vi "Configure Channels.vi"(8 "error in":errorcluster, 11 "Scope PXI CFG in":refnum<class "Scope PXI CFG.lvclass">) -> (0 "error out":errorcluster, 3 "Scope PXI CFG out":refnum<class "Scope PXI CFG.lvclass">)   [LabVIEW 2023, in "Scope.lvlib" / "Scope PXI.lvlib" / "Scope PXI CFG.lvclass"]
uses:
  Scope PXI CFG.lvclass
  D:/git/HAL/Configuration Base/Configuration Base.lvclass
  <instrlib>/niScope/Controls/niScope vertical coupling.ctl
  Scope PXI CFG.lvclass/Scope PXI CFG.ctl
  Configuration Base/Configuration Base.lvclass/Configuration Base.ctl
  853bd4bf-b846-4392-aaec-2eb0df7c15c1.vi
  fc1a35be-1af8-4cb9-88ab-84357ec016c8.vi
  c0a7b2a4-d6e1-41c5-8fb1-93d513341217.vi
  d2234409-928f-4ed9-b693-2867399abf4a.vi
  1e64d3fa-bcbf-4fb7-97e9-849c0281c434.vi
  2f0dfe3b-727d-435f-a334-361c3472aed8.vi
  a8bb4bbf-f82b-4e58-9fc0-885d6d8595a7.vi
  2afd0b27-f59c-4e4c-ab34-d1b063ee1579.vi
  46d73ebe-6710-4003-86ab-c95650fc7a2a.vi
  88285a36-7fea-47d7-9b3a-47c90033b7a9.vi
  <vilib>/JDP Science/JSONtext/Find Item.vi
  <vilib>/JDP Science/JSONtext/Next JSON Value.vi
  <vilib>/JDP Science/JSONtext/String Subset.vi
  <vilib>/JDP Science/JSONtext/Parsing/Advance past next JSON Value (inlined COPY).vi
  <vilib>/JDP Science/JSONtext/Parsing/Advance past whitespace.vi
  <vilib>/JDP Science/JSONtext/Parsing/Advance past String.vi
  <vilib>/JDP Science/JSONtext/Parsing/Advance past Number.vi
  <vilib>/JDP Science/JSONtext/Parsing/Advance past Line Ending.vi
  <vilib>/JDP Science/JSONtext/Parsing/Parse Full Path or Item Name.vi
  <vilib>/JDP Science/JSONtext/Parsing/Advance past Array.vi
  <vilib>/JDP Science/JSONtext/Parsing/Advance past Object.vi
  <vilib>/JDP Science/JSONtext/support/Error Cluster From Code.vi
  <vilib>/JDP Science/JSONtext/Offset/Find Item Locations by Path.vi
  <vilib>/JDP Science/JSONtext/JSON text to Variant.vi
  <vilib>/Utility/error.llb/Error Cluster From Error Code.vi
  <vilib>/JDP Science/JSONtext/LVClass Serializer/JSONtext LVClass Serializer.lvclass
  <vilib>/ErrorRing/Error Ring.xnode
  Configuration Base/Configuration Base.lvclass
panel:
  out "vertical coupling":T1=1 caption="vertical coupling (DC)" items=["AC", "DC", "Ground"]
  out "input impedance":u32(ring)=2 items=["1 mega ohm"=0, "50 ohms"=2]
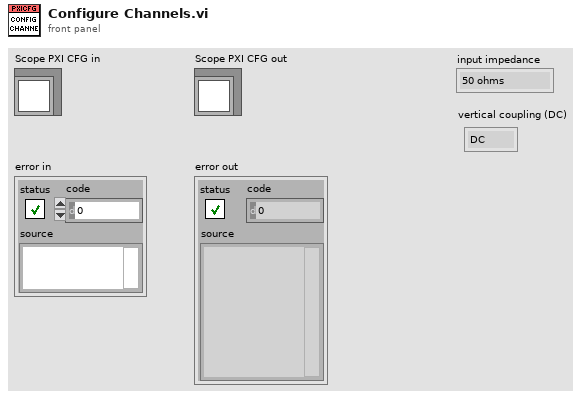
[diagram p1: front panel]
types:
  T1 = typedef "niScope vertical coupling.ctl" = i32
  T2 = typedef "LVStringsAndValuesArrayTypeDef_U32.ctl" = cluster{"String":string, "Value":u32}[]
  T3 = typedef "LVStringsAndValuesArrayTypeDef_I32.ctl" = cluster{"String":string, "Value":i32}[]
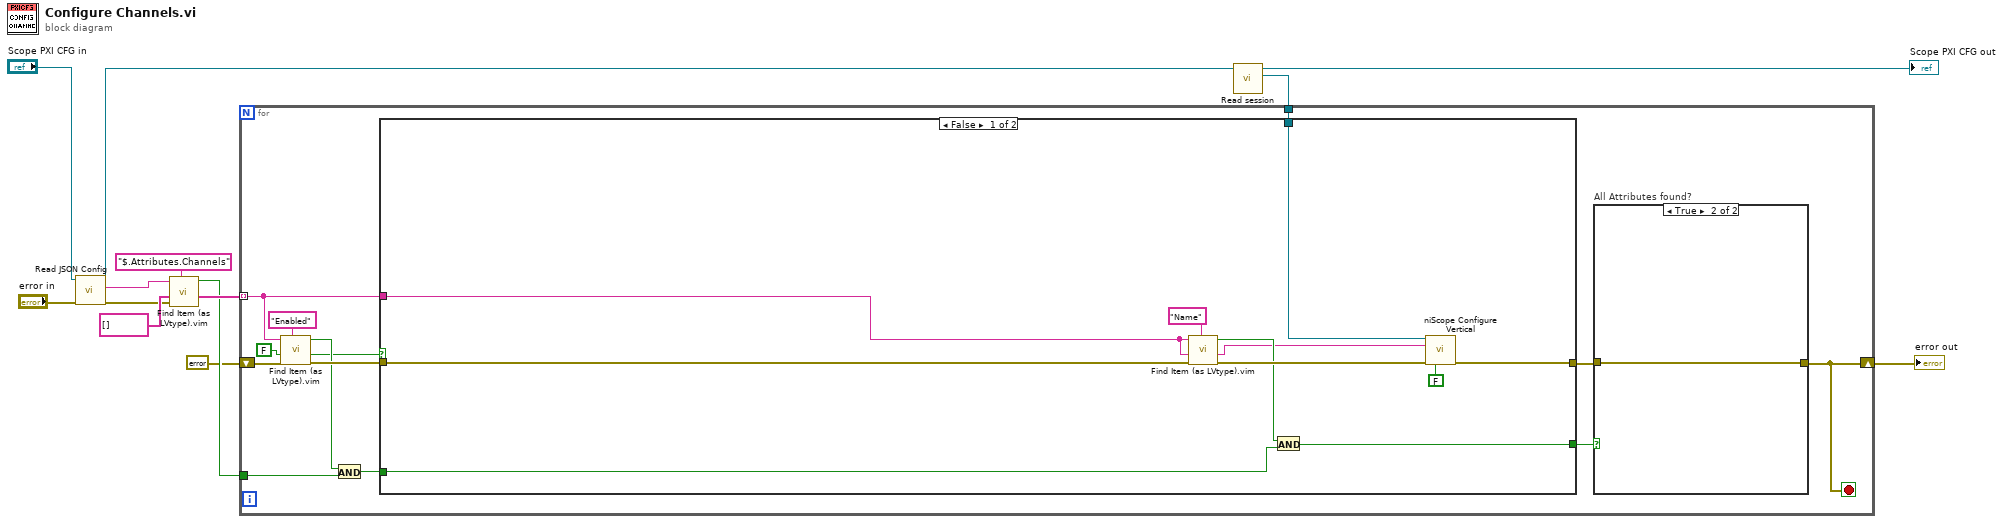
[diagram p0: block diagram]
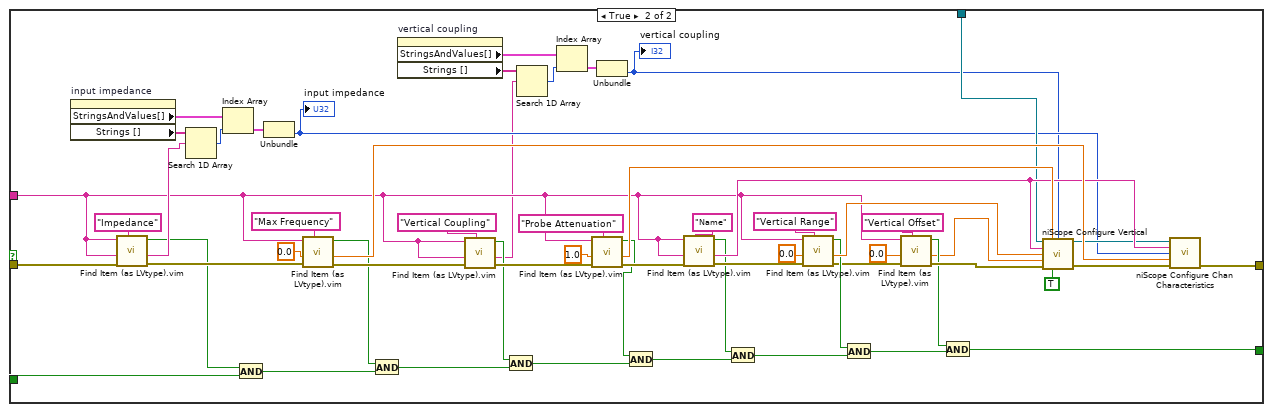
[diagram p2: hidden frame]
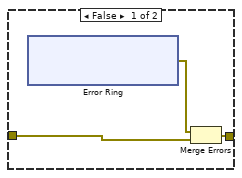
[diagram p3: hidden frame]
diagram:
  n1 = call "Read JSON Config.vi"("error in"="error in", "object in"="Scope PXI CFG in") -> ("error out"=w10:errorcluster, "<JSON>Config"=w11:string, "object out"=w2:refnum<class "Scope PXI CFG.lvclass">)  [unwired: 7 in]
  n2 = call "Find Item (as LVtype).vim"("$Path or Item Name"="$.Attributes.Channels", "error in (no error)"=w10, "Data Type and Default Value"=string[] [], "JSON"=w11) -> ("Data"=w9:string[], "Found"=w7:bool)  [unwired: 4 in, 2 out]
  n3 = call "Read session.vi"("Scope PXI CFG in"=w2) -> ("session"=w8:refnum<k15>, "Scope PXI CFG out"=→"Scope PXI CFG out":refnum<class "Scope PXI CFG.lvclass">)  [unwired: 8 in, 1 out]
  n4 = for {
    shift-right: [w14] -> w4
    shift-left: errorcluster {"status"=FALSE, "code"=0, "source"=""} ("error out") -> [w26]
    tunnel: w9 -> [w20] mode=indexing
    tunnel: w8 -> [w19]
    tunnel: w7 -> [w18]
    stop <- w14 stop-if-true
    n5 = call "Find Item (as LVtype).vim"("$Path or Item Name"="Enabled", "error in (no error)"=w26, "Data Type and Default Value"=FALSE, "JSON"=w20) -> ("error out"=w25:errorcluster, "Data"=w17:bool, "Found"=w22:bool)  [unwired: 4 in, 1 out]
    n6 = And(x=w22, y=w18) -> (x .and. y?=w23:bool)
    n7 = case shown="False" w17 {
      tunnel: [w27 w94] -> w16
      tunnel: w25 -> [w33 w77]
      tunnel: w23 -> [w37 w76]
      tunnel: w20 -> [w34 w44]
      tunnel: w19 -> [w28 w59]
      tunnel: [w31 w56] -> w15
      frame False {
        n8 = call "Find Item (as LVtype).vim"("$Path or Item Name"="Name", "error in (no error)"=w33, "Data Type and Default Value"=w34, "JSON"=w34) -> ("error out"=w32:errorcluster, "Data"=w29:string, "Found"=w30:bool)  [unwired: 4 in, 1 out]
        n9 = And(x=w30, y=w37) -> (x .and. y?=w31:bool)
        n10 = call <instrlib>:"niScope Configure Vertical.vi"("instrument handle"=w28, "channels"=w29, "error in"=w32, "channel enabled"=FALSE) -> ("error out"=w27:errorcluster)  [unwired: 10 in, 1 out]
      }
      frame True {
        n11 = property on="input impedance" class="Ring (strict)"() -> ("StringsAndValues[]"=w49:T2, "Strings []"=w48:string[])  [unwired: 2 in, 2 out]
        n12 = call "Find Item (as LVtype).vim"("$Path or Item Name"="Impedance", "error in (no error)"=w77, "Data Type and Default Value"=w44, "JSON"=w44) -> ("error out"=w93:errorcluster, "Data"=w47:string, "Found"=w46:bool)  [unwired: 4 in, 1 out]
        n13 = Search 1D Array(1D array=w48, element=w47) -> (index of element=w50:i32)  [unwired: 1 in]
        n14 = Index Array(array=w49, index=w50) -> (element=w51:cluster{"String":string, "Value":u32})
        n15 = And(x=w46, y=w76) -> (x .and. y?=w74:bool)
        n16 = Unbundle(w51) -> ("Value"=w45:u32)  [unwired: 1 out]
        "input impedance" <- w45
        n17 = call "Find Item (as LVtype).vim"("$Path or Item Name"="Max Frequency", "error in (no error)"=w93, "Data Type and Default Value"=0.0, "JSON"=w44) -> ("error out"=w90:errorcluster, "Data"=w85:dbl, "Found"=w75:bool)  [unwired: 4 in, 1 out]
        n18 = And(x=w75, y=w74) -> (x .and. y?=w72:bool)
        n19 = property on="vertical coupling" class="Ring (strict)"() -> ("StringsAndValues[]"=w40:T3, "Strings []"=w43:string[])  [unwired: 2 in, 2 out]
        n20 = call "Find Item (as LVtype).vim"("$Path or Item Name"="Vertical Coupling", "error in (no error)"=w90, "Data Type and Default Value"=w44, "JSON"=w44) -> ("error out"=w86:errorcluster, "Data"=w41:string, "Found"=w73:bool)  [unwired: 4 in, 1 out]
        n21 = And(x=w73, y=w72) -> (x .and. y?=w70:bool)
        n22 = Search 1D Array(1D array=w43, element=w41) -> (index of element=w42:i32)  [unwired: 1 in]
        n23 = Index Array(array=w40, index=w42) -> (element=w39:cluster{"String":string, "Value":i32})
        n24 = call "Find Item (as LVtype).vim"("$Path or Item Name"="Probe Attenuation", "error in (no error)"=w86, "Data Type and Default Value"=1.0, "JSON"=w44) -> ("error out"=w82:errorcluster, "Data"=w84:dbl, "Found"=w71:bool)  [unwired: 4 in, 1 out]
        n25 = Unbundle(w39) -> ("Value"=w38:i32)  [unwired: 1 out]
        "vertical coupling" <- w38
        n26 = And(x=w71, y=w70) -> (x .and. y?=w68:bool)
        n27 = call "Find Item (as LVtype).vim"("$Path or Item Name"="Name", "error in (no error)"=w82, "Data Type and Default Value"=w44, "JSON"=w44) -> ("error out"=w81:errorcluster, "Data"=w80:string, "Found"=w69:bool)  [unwired: 4 in, 1 out]
        n28 = And(x=w69, y=w68) -> (x .and. y?=w66:bool)
        n29 = call "Find Item (as LVtype).vim"("$Path or Item Name"="Vertical Range", "error in (no error)"=w81, "Data Type and Default Value"=0.0, "JSON"=w44) -> ("error out"=w63:errorcluster, "Data"=w78:dbl, "Found"=w67:bool)  [unwired: 4 in, 1 out]
        n30 = And(x=w67, y=w66) -> (x .and. y?=w65:bool)
        n31 = call "Find Item (as LVtype).vim"("$Path or Item Name"="Vertical Offset", "error in (no error)"=w63, "Data Type and Default Value"=0.0, "JSON"=w44) -> ("error out"=w62:errorcluster, "Data"=w60:dbl, "Found"=w61:bool)  [unwired: 4 in, 1 out]
        n32 = And(x=w61, y=w65) -> (x .and. y?=w56:bool)
        n33 = call <instrlib>:"niScope Configure Vertical.vi"("instrument handle"=w59, "probe attenuation"=w84, "vertical coupling"=w38, "channels"=w80, "vertical range"=w78, "vertical offset"=w60, "error in"=w62, "channel enabled"=TRUE) -> ("instrument handle out"=w53:refnum<k15>, "error out"=w55:errorcluster)  [unwired: 6 in]
        n34 = call <instrlib>:"niScope Configure Chan Characteristics.vi"("instrument handle"=w53, "channels"=w80, "input impedance"=w45, "maximum input frequency"=w85, "error in"=w55) -> ("error out"=w94:errorcluster)  [unwired: 9 in, 1 out]
      }
    }
    n35 = case "All Attributes found?" shown="True" w15 {
      tunnel: [w95 w103] -> w14
      tunnel: w16 -> [w96 w103]
      frame False {
        n36 = xnode "Error Ring"() -> ("error out"=w97:errorcluster)
        n37 = Merge Errors(w97, w96) -> (w95:errorcluster)
      }
      frame True {
      }
    }
  }
  "error out" <- w4
